vi "Sub - Arrow Point Calculate.vi"(0 "original position":cluster{"x":dbl, "y":dbl}, 2 "new position":cluster{"X":dbl, "Y":dbl}, 6 "tail length(10)":dbl=10.0, 8 "angle(30)":dbl=30.0) -> (14 "Tail endpoint 1":cluster{dbl, dbl}, 16 "Tail endpoint 2":cluster{dbl, dbl})   [LabVIEW 2015]
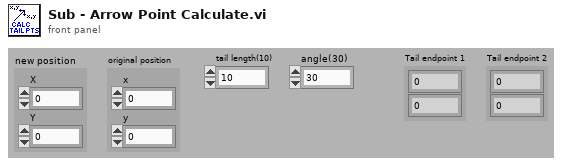
[diagram p1: front panel]
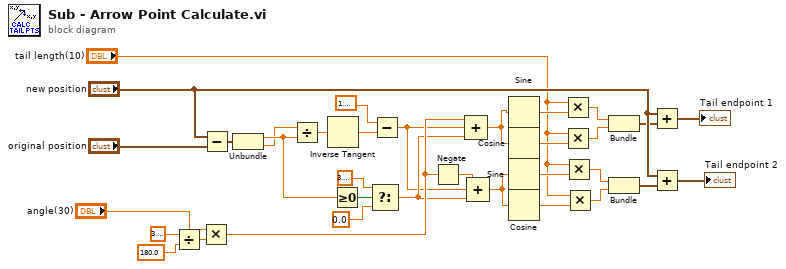
[diagram p0: block diagram]
diagram:
  n1 = Divide(x=3.141592653589793, y=180.0) -> (x/y=w31:dbl)
  n2 = Multiply(x="angle(30)", y=w31) -> (x*y=w32:dbl)
  n3 = Subtract(x="new position", y="original position") -> (x-y=w3:cluster{dbl, dbl})
  n4 = Unbundle(w3) -> (w23:dbl, w4:dbl)
  n5 = Divide(x=w4, y=w23) -> (x/y=w14:dbl)
  n6 = Inverse Tangent(1:w14) -> (0:w22:dbl)
  n7 = Greater Or Equal To 0?(x=w23) -> (x >= 0?=w13:bool)
  n8 = Select(t=3.141592653589793, s=w13, f=0.0) -> (s? t:f=w24:dbl)
  n9 = Subtract(x=1.5707963267948966, y=w22) -> (x-y=w21:dbl)
  n10 = Negate(x=w32) -> (-x=w28:dbl)
  n11 = Compound Arithmetic op=ADD(w32, w21, w24) -> (w7:dbl)
  n12 = Compound Arithmetic op=ADD(w28, w21, w24) -> (w19:dbl)
  n13 = Sine(x=w7) -> (sin(x)=w9:dbl)
  n14 = Cosine(x=w7) -> (cos(x)=w8:dbl)
  n15 = Sine(x=w19) -> (sin(x)=w17:dbl)
  n16 = Cosine(x=w19) -> (cos(x)=w18:dbl)
  n17 = Multiply(x="tail length(10)", y=w9) -> (x*y=w10:dbl)
  n18 = Multiply(x="tail length(10)", y=w8) -> (x*y=w11:dbl)
  n19 = Multiply(x="tail length(10)", y=w17) -> (x*y=w16:dbl)
  n20 = Multiply(x="tail length(10)", y=w18) -> (x*y=w15:dbl)
  n21 = Bundle(w10, w11) -> (w5:cluster{dbl, dbl})  [unwired: 1 in]
  n22 = Bundle(w16, w15) -> (w20:cluster{dbl, dbl})  [unwired: 1 in]
  n23 = Add(x="new position", y=w5) -> (x+y=→"Tail endpoint 1":cluster{dbl, dbl})
  n24 = Add(x="new position", y=w20) -> (x+y=→"Tail endpoint 2":cluster{dbl, dbl})
